vi "GetSystemParameterInteger.vi"(8 "error in (no error)":errorcluster, 9 "Parameter Name":string(combo), 11 "controller in":refnum<k24>) -> (0 "error out":errorcluster, 2 "value":i32, 3 "controller out":refnum<k24>)   [LabVIEW 2020, in "Aerotech.lvlib"]
uses:
  Aerotech.lvlib
  C:/Users/HEP/Documents/GitHub/UCSB-Gantry-HEP/Drivers/Aerotech A3200/Bin/Aerotech.A3200.LabVIEW.dll
  UCSB-Gantry-HEP/Drivers/Aerotech A3200/Bin/Aerotech.A3200.LabVIEW.dll
  C:/Program Files (x86)/Aerotech/A3200/LabVIEW/2010/Bin/Aerotech.A3200.dll
  Program Files (x86)/Aerotech/A3200/LabVIEW/2010/Bin/Aerotech.A3200.dll
panel:
  out "ParameterType":i32(ring) items=["Integer", "Double", "Single", "Long", "String"]
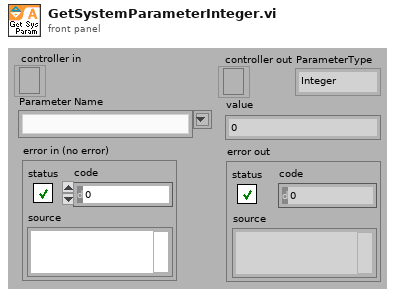
[diagram p1: front panel]
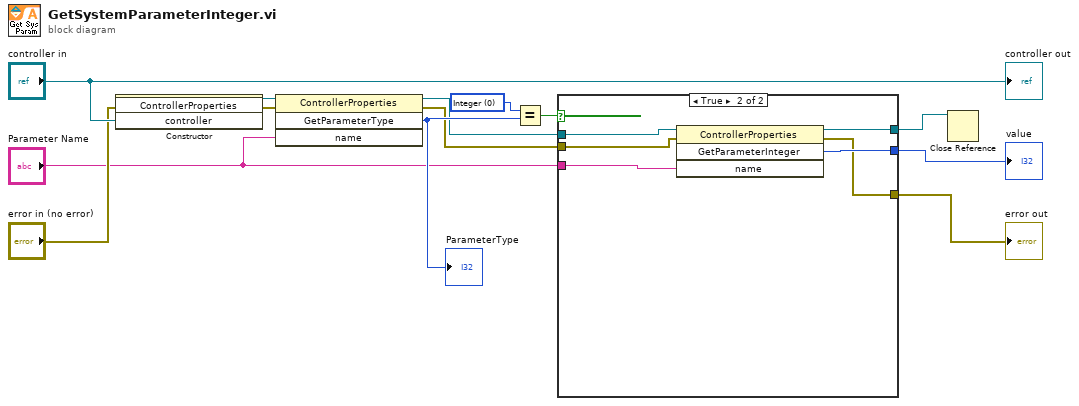
[diagram p0: block diagram]
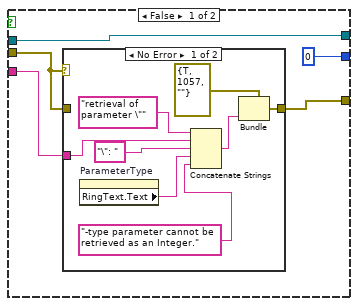
[diagram p2: hidden frame]
diagram:
  w9 = 0 items=["Integer", "Double", "Single", "Long", "String"] ("GetParameterType")
  n1 = constructor class="ControllerProperties"(error in="error in (no error)", "controller"="controller in") -> (reference out=w11:refnum<k24>, error out=w10:errorcluster)  [unwired: 2 in, 2 out]
  n2 = invoke class="ControllerProperties" method="GetParameterType"(reference=w11, error in=w10, "name"="Parameter Name") -> (reference out=w5:refnum<k24>, error out=w4:errorcluster, "GetParameterType"=w8:i32)  [unwired: 1 in, 1 out]
  "ParameterType" <- w8
  n3 = Equal?(x=w9, y=w8) -> (x = y?=w7:bool)
  n4 = case shown="True" w7 {
    tunnel: [w18 w32] -> w6
    tunnel: w5 -> [w18 w33]
    tunnel: "Parameter Name" -> [w14 w31]
    tunnel: w4 -> [w15 w30]
    tunnel: [0 w29] -> w3
    tunnel: [w16 w28] -> w2
    frame False {
      n5 = case shown="No Error" w15 {
        tunnel: [w25 w27] -> w16
        tunnel: w15 -> [_ w27]
        tunnel: w14 -> [w22 _]
        frame No Error {
          n6 = property on="ParameterType" class="Ring (strict)"() -> ("RingText.Text"=w20:string)  [unwired: 2 in, 2 out]
          n7 = Concatenate Strings("retrieval of parameter \"" ("string"), w22, "\": " ("string"), w20, "-type parameter cannot be retrieved as an Integer." ("string")) -> (w24:string)
          n8 = Bundle(cluster=cluster{bool, "code":i32, "source":string} {TRUE, "code"=1057, "source"=""} ("error out"), "source"=w24) -> (w25:cluster{bool, "code":i32, "source":string})  [unwired: 2 in]
        }
        frame Error {
        }
      }
    }
    frame True {
      n9 = invoke class="ControllerProperties" method="GetParameterInteger"(reference=w33, error in=w30, "name"=w31) -> (reference out=w32:refnum<k24>, error out=w28:errorcluster, "GetParameterInteger"=w29:i32)  [unwired: 1 in, 1 out]
    }
  }
  "error out" <- w2
  "value" <- w3
  n10 = Close Reference(reference=w6) -> ()  [unwired: 1 in, 1 out]
  "controller out" <- "controller in"
